vi "LeastSquareCalculation.vi"(6 "array 4":dbl[](array[numeric]), 9 "array 3":dbl[](array[numeric]), 10 "array 2":dbl[](array[numeric]), 11 "array":dbl[](array[numeric])) -> (3 "Numeric":dbl)   [LabVIEW 2013]
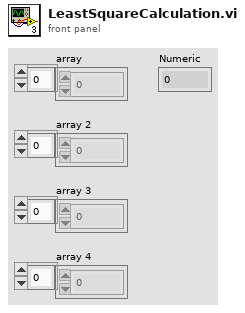
[diagram p1: front panel]
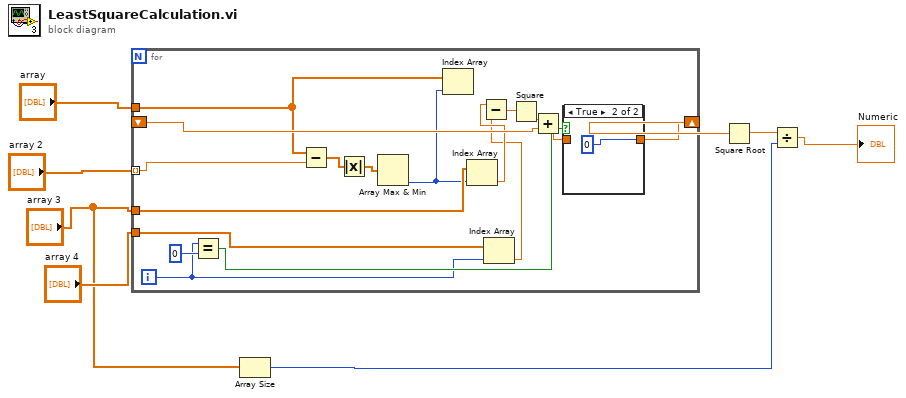
[diagram p0: block diagram]
diagram:
  n1 = for {
    tunnel: "array 2" -> [w20] mode=indexing
    shift-right: [w16] -> w5
    shift-left: _ -> [w21]
    tunnel: "array" -> [w19]
    tunnel: "array 4" -> [w14]
    tunnel: "array 3" -> [w13]
    i -> [w9]
    n2 = Equal?(x=w9, y=0) -> (x = y?=w17:bool)
    n3 = Subtract(x=w19, y=w20) -> (x-y=w25:dbl[])
    n4 = Absolute Value(x=w25) -> (abs(x)=w24:dbl[])
    n5 = Array Max & Min(array=w24) -> (min index (indices)=w12:i32)  [unwired: 3 out]
    n6 = Index Array(array=w19, index=w12) -> ()  [unwired: 1 out]
    n7 = Index Array(array=w13, index=w12) -> (element=w11:dbl)
    n8 = Index Array(array=w14, index=w9) -> (element=w10:dbl)
    n9 = Subtract(x=w11, y=w10) -> (x-y=w23:dbl)
    n10 = Square(x=w23) -> (x^2=w22:dbl)
    n11 = Add(x=w22, y=w21) -> (x+y=w15:dbl)
    n12 = case shown="True" w17 {
      tunnel: [w26 0 ("y")] -> w16
      tunnel: w15 -> [w26 _]
      frame False {
      }
      frame True {
      }
    }
  }
  n13 = Array Size(array="array 3") -> (size(s)=w1:i32)
  n14 = Square Root(x=w5) -> (sqrt(x)=w3:dbl)
  n15 = Divide(x=w3, y=w1) -> (x/y=→"Numeric":dbl)
